vi "Send Command.vi"(8 "error in":errorcluster, 9 "Value":variant, 10 "Command":string, 11 "MLTFNC in":refnum<class "MLTFNC.lvclass">) -> (0 "error out":errorcluster, 3 "MLTFNC out":refnum<class "MLTFNC.lvclass">)   [LabVIEW 2019, in "MLTFNC.lvlib" / "MLTFNC.lvclass"]
uses:
  Library/MLTFNC.lvclass
  C:/Users/Public/Documents/Development/builds/Engine/Engine.lvlibp/Project/Engine.lvclass
  MLTFNC Messages/Toggle Channel Msg/Toggle Channel Msg.lvclass/Toggle Channel Msg.ctl
  builds/Engine/Engine.lvlibp/Accessors/Read Self Q.vi
  builds/Engine/Actor Framework.lvlibp/1abvi3w/vi.lib/ActorFramework/Message Enqueuer/Enqueue.vi
  builds/Engine/Actor Framework.lvlibp/1abvi3w/vi.lib/ActorFramework/Message Enqueuer/Message Enqueuer.lvclass
  MLTFNC Messages/Toggle Channel Msg/Toggle Channel Msg.lvclass
  MLTFNC Messages/Clear All Msg/Clear All Msg.lvclass
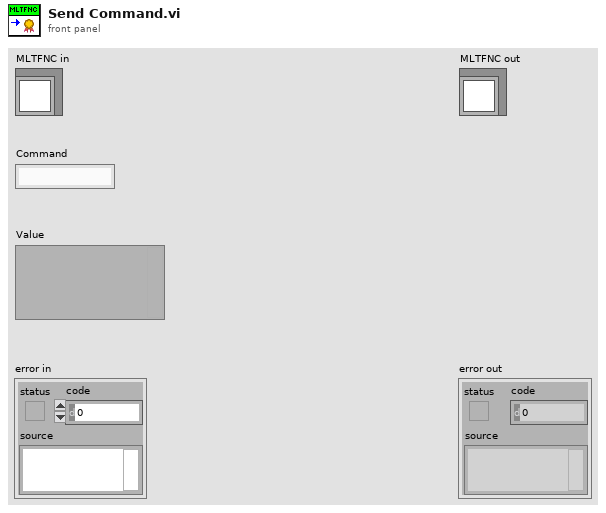
[diagram p1: front panel]
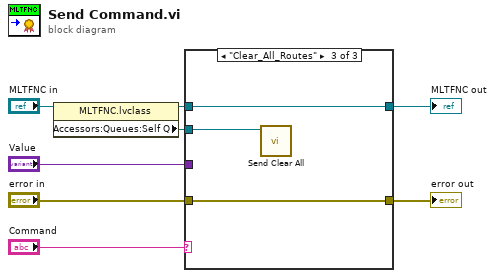
[diagram p0: block diagram]
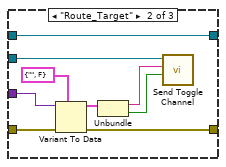
[diagram p3: hidden frame]
diagram:
  n1 = property class="MLTFNC.lvclass"(reference="MLTFNC in") -> (reference out=w2:refnum<class "MLTFNC.lvclass">, "Accessors:Queues:Self Q"=w1:refnum<class "Message Enqueuer.lvclass">)  [unwired: 1 in, 1 out]
  n2 = case shown="\"Clear_All_Routes\"" "Command" {
    tunnel: w2 -> [w10 w15 w22]
    tunnel: [w10 w15 w22] -> w6
    tunnel: "error in" -> [w9 w19 w20]
    tunnel: [w9 w14 w20] -> w4
    tunnel: "Value" -> [_ w18 _]
    tunnel: w1 -> [_ w13 w21]
    frame Default {
    }
    frame "Route_Target" {
      n3 = Variant To Data(error in=w19, type=cluster{"Target":string, "Connect":bool} {"Target"="", "Connect"=FALSE}, Variant=w18) -> (data=w16:cluster{"Target":string, "Connect":bool}, error out=w14:errorcluster)
      n4 = Unbundle(w16) -> ("Target"=w12:string, "Connect"=w11:bool)
      n5 = call "Send Toggle Channel.vi"("State"=w11, "Name"=w12, "Message Enqueuer"=w13) -> ()  [unwired: 7 in, 2 out]
    }
    frame "Clear_All_Routes" {
      n6 = call "Send Clear All.vi"("Message Enqueuer"=w21) -> ()  [unwired: 9 in, 2 out]
    }
  }
  "error out" <- w4
  "MLTFNC out" <- w6
